vi "Get Case Insensitive Search Pattern.vi"(2 "case matching (sensitive)":T1=enum."system", 3 "regular expression":string) -> (1 "case insensitive regular expression":string)   [LabVIEW 2012, in "Car Wash.lvlib" / "Tools_String.lvlib"]
doc: "Changes a regular expression (used by Match Pattern) to perform a case insensitive match.\n\nWhen match case is TRUE, the regular expression will not be changed."
uses:
  Tools_String.lvlib
  <vilib>/FTP/util/Case Matching.ctl
  <vilib>/FTP/NI_FTP.lvlib
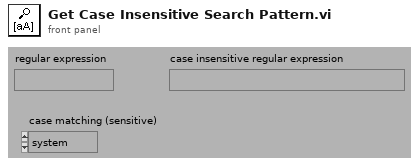
[diagram p1: front panel]
types:
  T1 = typedef "NI_FTP.lvlib/Case Matching.ctl" = enum16{"a != A", "a == A", "system"}
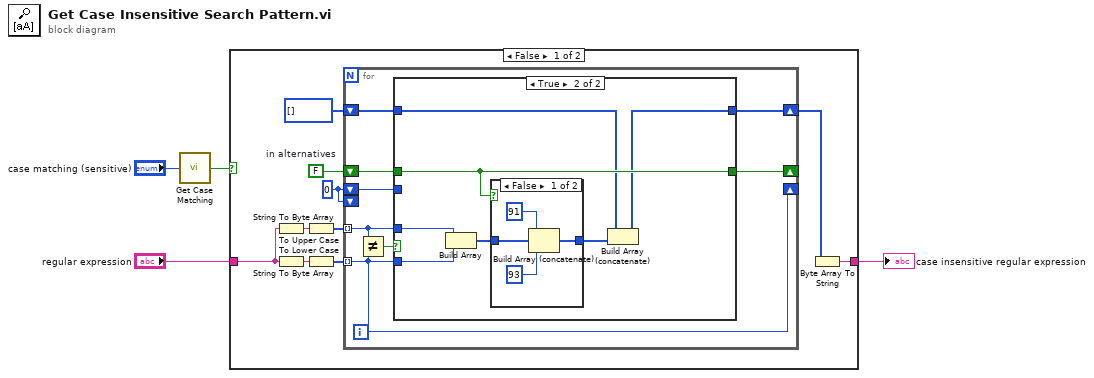
[diagram p0: block diagram]
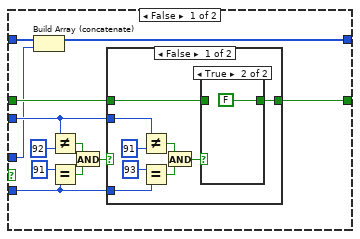
[diagram p2: hidden frame]
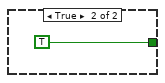
[diagram p4: hidden frame]
diagram:
  n1 = call "Get Case Matching.vi"("string matching"="case matching (sensitive)") -> ("match case"=w1:bool)
  n2 = case shown="False" w1 {
    tunnel: "regular expression" -> [w8 w59]
    tunnel: [w7 w59] -> w4
    frame False {
      w14 = u8 0
      w13 = FALSE  # in alternatives
      n3 = To Upper Case(1:w8) -> (0:w11:string)
      n4 = To Lower Case(string=w8) -> (all lower case string=w12:string)
      n5 = String To Byte Array(string=w11) -> (unsigned byte array=w10:u8[])
      n6 = String To Byte Array(string=w12) -> (unsigned byte array=w9:u8[])
      n7 = for {
        shift-right: [w18] -> w6
        shift-left: u8[] [] -> [w19]
        tunnel: w9 -> [w16] mode=indexing
        tunnel: w10 -> [w15] mode=indexing
        shift-right: [w16] -> _
        shift-left: w14 -> [w17]
        shift-right: [w22] -> _
        shift-left: w13 -> [w21]
        shift-left: w14 -> [_]
        n8 = Not Equal?(x=w15, y=w16) -> (x != y?=w20:bool)
        n9 = case shown="True" w20 {
          tunnel: w17 -> [w24 _]
          tunnel: [w33 w53] -> w22
          tunnel: w21 -> [w32 w53]
          tunnel: w16 -> [w30 w52]
          tunnel: w19 -> [w26 w49]
          tunnel: [w25 w48] -> w18
          tunnel: w15 -> [w23 w47]
          frame False {
            n10 = Build Array (concatenate)(w26, w23) -> (w25:u8[])
            n11 = Not Equal?(x=w24, y=u8 92) -> (x != y?=w29:bool)
            n12 = Equal?(x=u8 91, y=w30) -> (x = y?=w28:bool)
            n13 = And(x=w29, y=w28) -> (x .and. y?=w27:bool)
            n14 = case shown="False" w27 {
              tunnel: [w41 TRUE] -> w33
              tunnel: w32 -> [w43 _]
              tunnel: w30 -> [w40 _]
              tunnel: w24 -> [w42 _]
              frame False {
                n15 = Not Equal?(x=w42, y=u8 91) -> (x != y?=w36:bool)
                n16 = Equal?(x=u8 93, y=w40) -> (x = y?=w37:bool)
                n17 = And(x=w36, y=w37) -> (x .and. y?=w35:bool)
                n18 = case shown="True" w35 {
                  tunnel: w43 -> [w44 _]
                  tunnel: [w44 FALSE ("in alternatives")] -> w41
                  frame False {
                  }
                  frame True {
                  }
                }
              }
              frame True {
              }
            }
          }
          frame True {
            n19 = Build Array(w47, w52) -> (w51:u8[])
            n20 = case shown="False" w53 {
              tunnel: w51 -> [w57 w58]
              tunnel: [w56 w58] -> w50
              frame False {
                n21 = Build Array (concatenate)(u8 91, w57, u8 93) -> (w56:u8[])
              }
              frame True {
              }
            }
            n22 = Build Array (concatenate)(w49, w50) -> (w48:u8[])
          }
        }
      }
      n23 = Byte Array To String(unsigned byte array=w6) -> (string=w7:string)
    }
    frame True {
    }
  }
  "case insensitive regular expression" <- w4
